vi "UDP Send.vi"   [LabVIEW 2013]
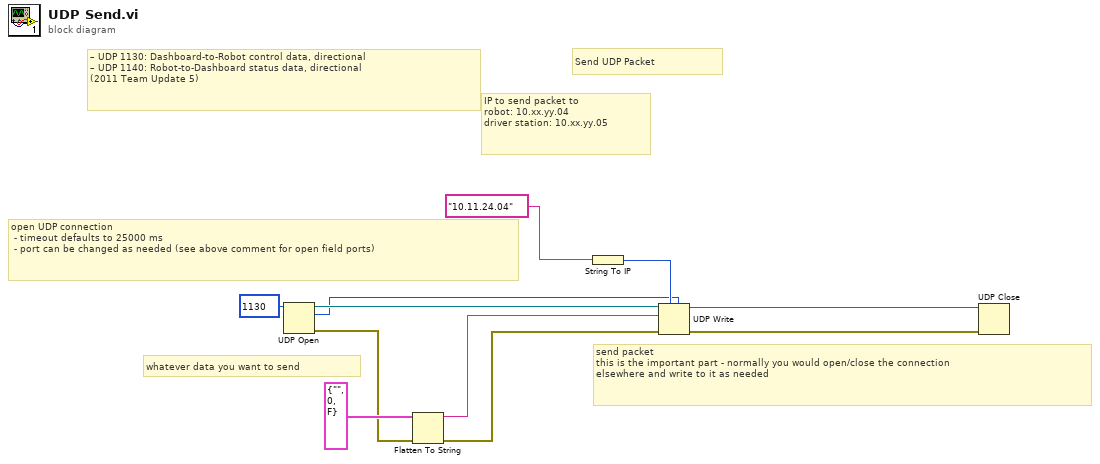
[diagram p0: block diagram]
diagram:
  # "send packet\nthis is the important part - normally you would open/close the connection \nelsewhere and write to it as needed"
  # "whatever data you want to send"
  # "IP to send packet to \nrobot: 10.xx.yy.04\ndriver station: 10.xx.yy.05"
  # "open UDP connection\n - timeout defaults to 25000 ms\n - port can be changed as needed (see above comment for open field ports)"
  # "Send UDP Packet"
  # "– UDP 1130: Dashboard-to-Robot control data, directional\n– UDP 1140: Robot-to-Dashboard status data, directional\n(2011 Team Update 5)"
  n1 = UDP Open(11:u16 1130 ("port")) -> (port=w10:refnum<k16>, 0:w5:errorcluster, 2:w7:u16)  [unwired: 1 in, 3 out]
  n2 = Flatten To String(anything=cluster{string, i32, bool} {"", 0, FALSE}, error in (no error)=w5) -> (data string=w3:string, error out=w4:errorcluster)  [unwired: 3 out]
  n3 = String To IP(1:"10.11.24.04") -> (0:w8:u32)
  n4 = UDP Write(address=w8, port or service name=w7, connection ID=w10, data in=w3, 8:w4) -> (error out=w1:errorcluster, 3:w2:refnum<k16>)  [unwired: 1 out]
  n5 = UDP Close(connection ID=w2, 8:w1) -> ()  [unwired: 2 out]
